vi "SICMExperimentOnCheck.vi"(8 "error in (no error)":errorcluster, 11 "Refnum in":T1) -> (0 "error out":errorcluster, 1 "IsExperimentSICM?":bool, 3 "Refnum out":T1)   [LabVIEW 2016]
uses:
  controls/FPGAVIreferenceTypeDef.ctl
  <vilib>/Utility/error.llb/Error Cluster From Error Code.vi
  <vilib>/rvi/errors/niLvFpgaAdjustHostInterfaceError.vi
  <vilib>/rvi/interface/nirviReadWriteControl/nirviReadWriteControl.xnode
  FPGA Bitfiles/qnmController797_usbRIO_controllerFPGAmu.lvbitx
  NiFpgaLv.dll
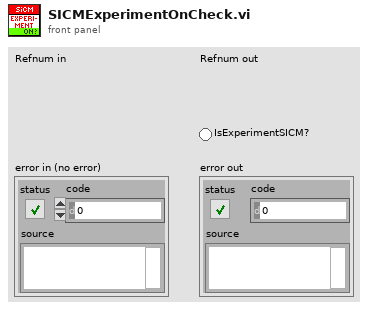
[diagram p1: front panel]
types:
  T1 = typedef "FPGAVIreferenceTypeDef.ctl" = refnum<k20>
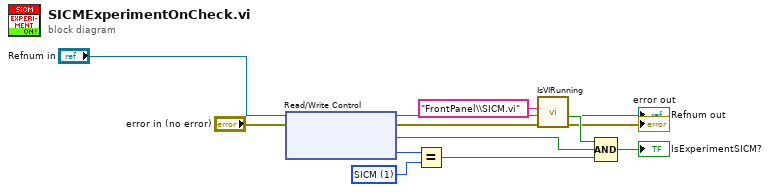
[diagram p0: block diagram]
diagram:
  w10 = u8 1 items=["process Variable", "SICM"] ("flt.i.bypassSource")
  n1 = xnode "Read/Write Control"("FPGA VI Reference In"="Refnum in", "error in"="error in (no error)") -> ("FPGA VI Reference Out"=→"Refnum out":T1, "error out"=w5:errorcluster, "flt.bypassPI"=w12:bool, "flt.i.bypassSource"=w9:u8)
  n2 = Equal?(x=w9, y=w10) -> (x = y?=w11:bool)
  n3 = call "IsVIRunning.vi"("error in (no error)"=w5, "name or relative path"="FrontPanel\\SICM.vi") -> ("error out"=→"error out":errorcluster, "RunningVI?"=w7:bool)  [unwired: 8 in]
  n4 = Compound Arithmetic op=AND(w7, w12, w11) -> (→"IsExperimentSICM?":bool)
